vi "sys_info.vi"(9 "枚举":enum16{"write", "read"}(ring)=enum."read", 11 "sys_info":string) -> (3 "sys_info":string)   [LabVIEW 2018]
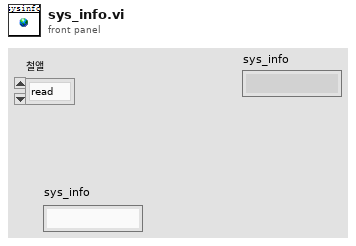
[diagram p1: front panel]
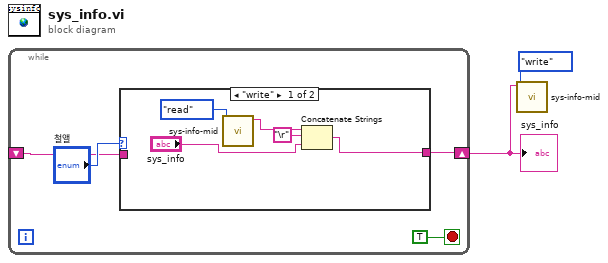
[diagram p0: block diagram]
diagram:
  n1 = while {
    shift-right: [w4] -> w2
    shift-left: _ -> [w3]
    stop <- TRUE stop-if-true
    n2 = case shown="\"write\"" "枚举" {
      tunnel: [w7 w12] -> w4
      tunnel: w3 -> [_ w12]
      frame "write" {
        n3 = call "sys-info-mid.vi"("枚举"=enum16{"write", "read"}."read") -> ("info"=w10:string)  [unwired: 10 in]
        n4 = Concatenate Strings(w10, "\r", "sys_info") -> (w7:string)
      }
      frame "read", Default {
      }
    }
  }
  "sys_info" <- w2
  n5 = call "sys-info-mid.vi"("枚举"=enum16{"write", "read"}."write", "info"=w2) -> ()  [unwired: 9 in, 1 out]
